vi "RPM_SubVI.vi"(0 "High Byte":u8, 3 "Low Byte":u8) -> (7 "RPM":dbl)   [LabVIEW 2012]
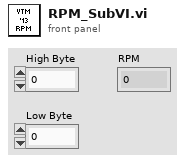
[diagram p1: front panel]
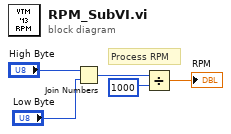
[diagram p0: block diagram]
diagram:
  # "Process RPM"
  n1 = Join Numbers(hi="High Byte", lo="Low Byte") -> ((hi.lo)=w3:u16)
  n2 = Divide(x=w3, y=u16 1000) -> (x/y=→"RPM":dbl)
